vi "scaling_map.vi"(8 "m_b":dbl[](array[numeric]), 11 "x":dbl) -> (2 "y":dbl)   [LabVIEW 2017]
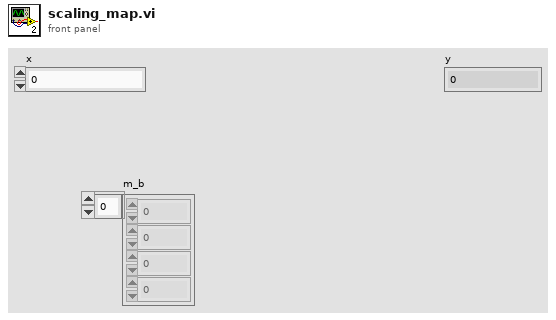
[diagram p1: front panel]
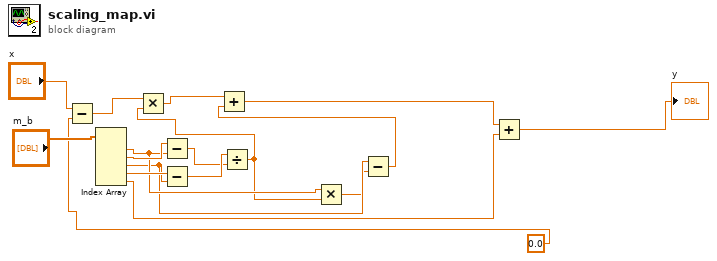
[diagram p0: block diagram]
diagram:
  n1 = Subtract(x="x", y=0.0) -> (x-y=w3:dbl)
  n2 = Index Array(array="m_b") -> (element #1=w11:dbl, element #2=w15:dbl, element #3=w9:dbl, element #4=w14:dbl, element #5=w2:dbl)  [unwired: 5 in]
  n3 = Subtract(x=w15, y=w11) -> (x-y=w12:dbl)
  n4 = Subtract(x=w14, y=w9) -> (x-y=w13:dbl)
  n5 = Divide(x=w13, y=w12) -> (x/y=w10:dbl)
  n6 = Multiply(x=w3, y=w10) -> (x*y=w17:dbl)
  n7 = Multiply(x=w11, y=w10) -> (x*y=w8:dbl)
  n8 = Subtract(x=w9, y=w8) -> (x-y=w7:dbl)
  n9 = Add(x=w17, y=w7) -> (x+y=w6:dbl)
  n10 = Add(x=w6, y=w2) -> (x+y=→"y":dbl)
